vi "NS Capacitance of Analyte Molecule.vi"(6 "Dielectric of Molecule Analyte":dbl, 7 "Molecule Length":dbl, 8 "# of CNTs":dbl, 9 "Surface Area 1 NS":dbl, 10 "Surface Area of 1 CNT":dbl, 11 "Permitivity of Free Space":dbl) -> (1 "Capaciatance per CNT":dbl, 2 "Capacitance Functional Analyte per NS":dbl, 3 "Capacitance Functional Analyte per NS 2":dbl, 4 "Capacitance Functinal Analyte  per unit area":dbl)   [LabVIEW 2020]
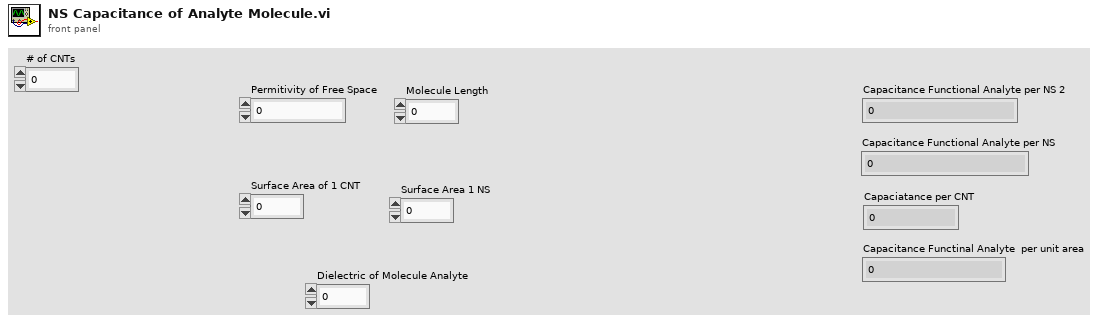
[diagram p1: front panel]
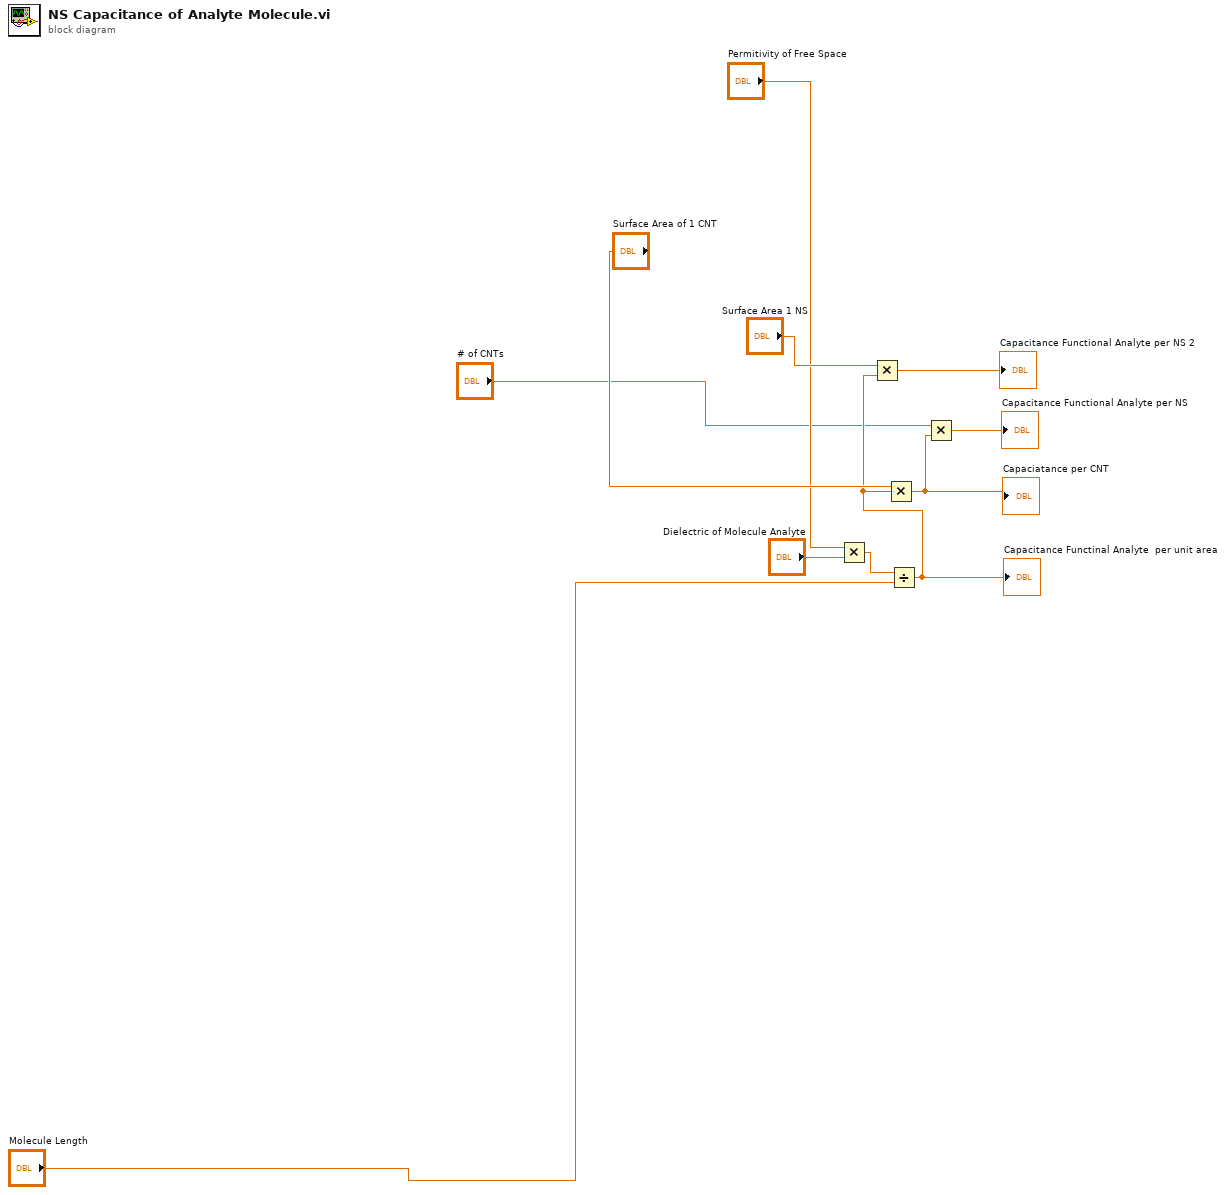
[diagram p0: block diagram]
diagram:
  n1 = Multiply(x="Permitivity of Free Space", y="Dielectric of Molecule Analyte") -> (x*y=w3:dbl)
  n2 = Divide(x=w3, y="Molecule Length") -> (x/y=w6:dbl)
  "Capacitance Functinal Analyte  per unit area" <- w6
  n3 = Multiply(x="Surface Area 1 NS", y=w6) -> (x*y=→"Capacitance Functional Analyte per NS 2":dbl)
  n4 = Multiply(x="Surface Area of 1 CNT", y=w6) -> (x*y=w7:dbl)
  "Capaciatance per CNT" <- w7
  n5 = Multiply(x="# of CNTs", y=w7) -> (x*y=→"Capacitance Functional Analyte per NS":dbl)
